vi "Limelight Tank.vi"() -> (10 "SteerCommand":dbl(knob)=0.28422717771668365 scale=-1.0..1.0, 11 "DriveCommand":dbl(knob)=-0.025869879478955773 scale=0.0..1.0)   [LabVIEW 2019]
uses:
  <vilib>/Rock Robotics/Network Tables/NT Read Number.vi
  Framework/Robot Global Data.vi
panel:
  out "Limelight Goal Area":dbl(slide)=1.91 min=0.1 max=2.5 step=0.25 scale=0.0..2.5
  out "TargetValid":bool=TRUE
  out "MaxDrive":dbl(slide)=0.6824817518248175 min=0.0 max=1.0 step=0.01 scale=0.0..1.0
  out "DriveK":dbl(slide)=0.26277372262773724 min=0.0 max=1.0 step=0.05 scale=0.0..1.0
  out "AimDeadband":dbl min=0.0 max=10.0 step=0.25
  out "MinSteerCommand":dbl(slide)=0.2 min=0.0 max=0.5 step=0.05 scale=0.0..0.5
  out "SteeringK":dbl(slide)=0.025362318840579712 min=0.0 max=0.25 step=0.01 scale=0.0..0.25
  # "0.271739"
  # "0.682482"
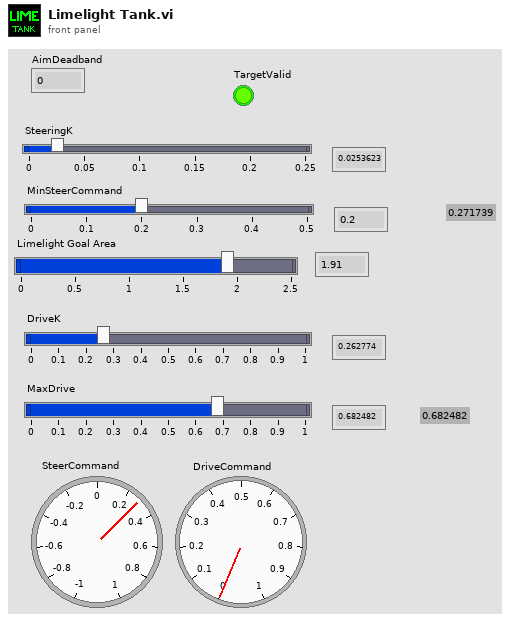
[diagram p1: front panel]
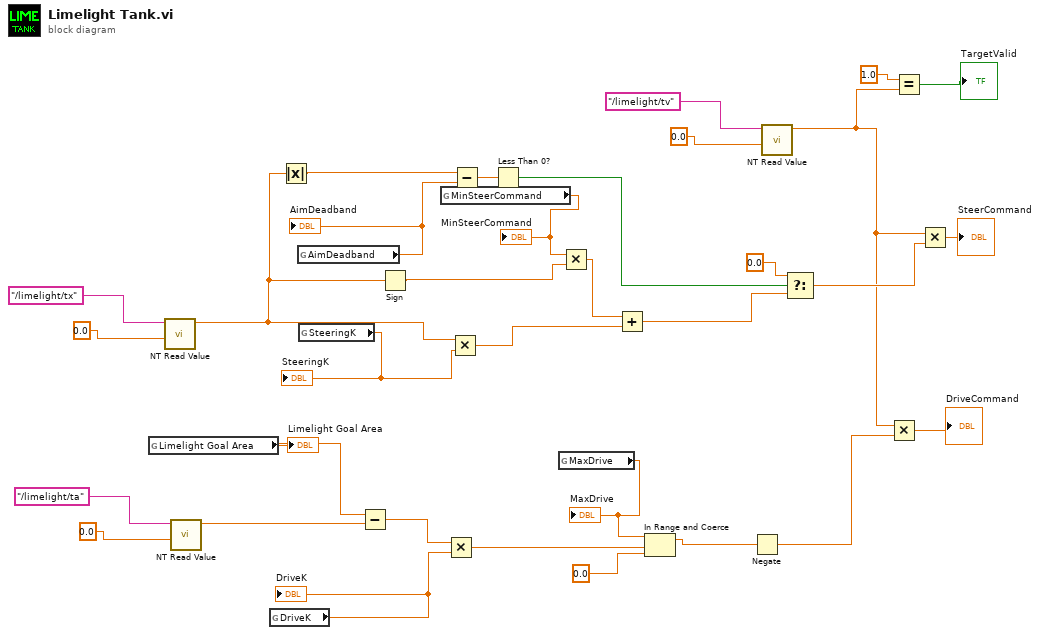
[diagram p0: block diagram]
diagram:
  n1 = global read "Robot Global Data.vi" "Limelight Goal Area"() -> (w6:dbl)
  "Limelight Goal Area" <- w6
  n2 = call-poly <vilib>:"NT Read Value.vi"("Default Value"=0.0, "Name"="/limelight/tx") -> ("Numeric"=w11:dbl)  [unwired: 8 in, 1 out]
  n3 = call-poly <vilib>:"NT Read Value.vi"("Default Value"=0.0, "Name"="/limelight/ta") -> ("Numeric"=w18:dbl)  [unwired: 8 in, 1 out]
  n4 = global read "Robot Global Data.vi" "DriveK"() -> (w2:dbl)
  "DriveK" <- w2
  n5 = Absolute Value(x=w11) -> (abs(x)=w30:dbl)
  n6 = global read "Robot Global Data.vi" "AimDeadband"() -> (w4:dbl)
  "AimDeadband" <- w4
  n7 = global read "Robot Global Data.vi" "SteeringK"() -> (w1:dbl)
  "SteeringK" <- w1
  n8 = Subtract(x=w6, y=w18) -> (x-y=w17:dbl)
  n9 = Sign(1:w11) -> (0:w19:dbl)
  n10 = global read "Robot Global Data.vi" "MinSteerCommand"() -> (w3:dbl)
  "MinSteerCommand" <- w3
  n11 = Multiply(x=w17, y=w2) -> (x*y=w16:dbl)
  n12 = Multiply(x=w11, y=w1) -> (x*y=w28:dbl)
  n13 = Subtract(x=w30, y=w4) -> (x-y=w31:dbl)
  n14 = Less Than 0?(x=w31) -> (x < 0?=w32:bool)
  n15 = global read "Robot Global Data.vi" "MaxDrive"() -> (w5:dbl)
  "MaxDrive" <- w5
  n16 = Multiply(x=w3, y=w19) -> (x*y=w29:dbl)
  n17 = Add(x=w29, y=w28) -> (x+y=w10:dbl)
  n18 = In Range and Coerce(upper limit=w5, x=w16, lower limit=0.0) -> (coerced(x)=w13:dbl)  [unwired: 1 out]
  n19 = Negate(x=w13) -> (-x=w12:dbl)
  n20 = call-poly <vilib>:"NT Read Value.vi"("Default Value"=0.0, "Name"="/limelight/tv") -> ("Numeric"=w9:dbl)  [unwired: 8 in, 1 out]
  n21 = Select(t=0.0, s=w32, f=w10) -> (s? t:f=w21:dbl)
  n22 = Multiply(x=w9, y=w12) -> (x*y=→"DriveCommand":dbl)
  n23 = Equal?(x=1.0, y=w9) -> (x = y?=→"TargetValid":bool)
  n24 = Multiply(x=w9, y=w21) -> (x*y=→"SteerCommand":dbl)
